vi "Reading HTML.vi"() -> ()   [LabVIEW 2024]
uses:
  <vilib>/httpClient/POSTBuffer.vi
  <vilib>/httpClient/LabVIEWHTTPClient.lvlib
panel:
  out "headers 3":string
  out "body 3":string
  out "headers 2":string
  out "body 2":string
  in  "Pulse number 2":string="5"
  out "body":string="{\"message\":\"success\"}"
  out "headers":string="HTTP/1.1 200 OK\r\nTransfer-Encoding: chunked\r\n\r\n"
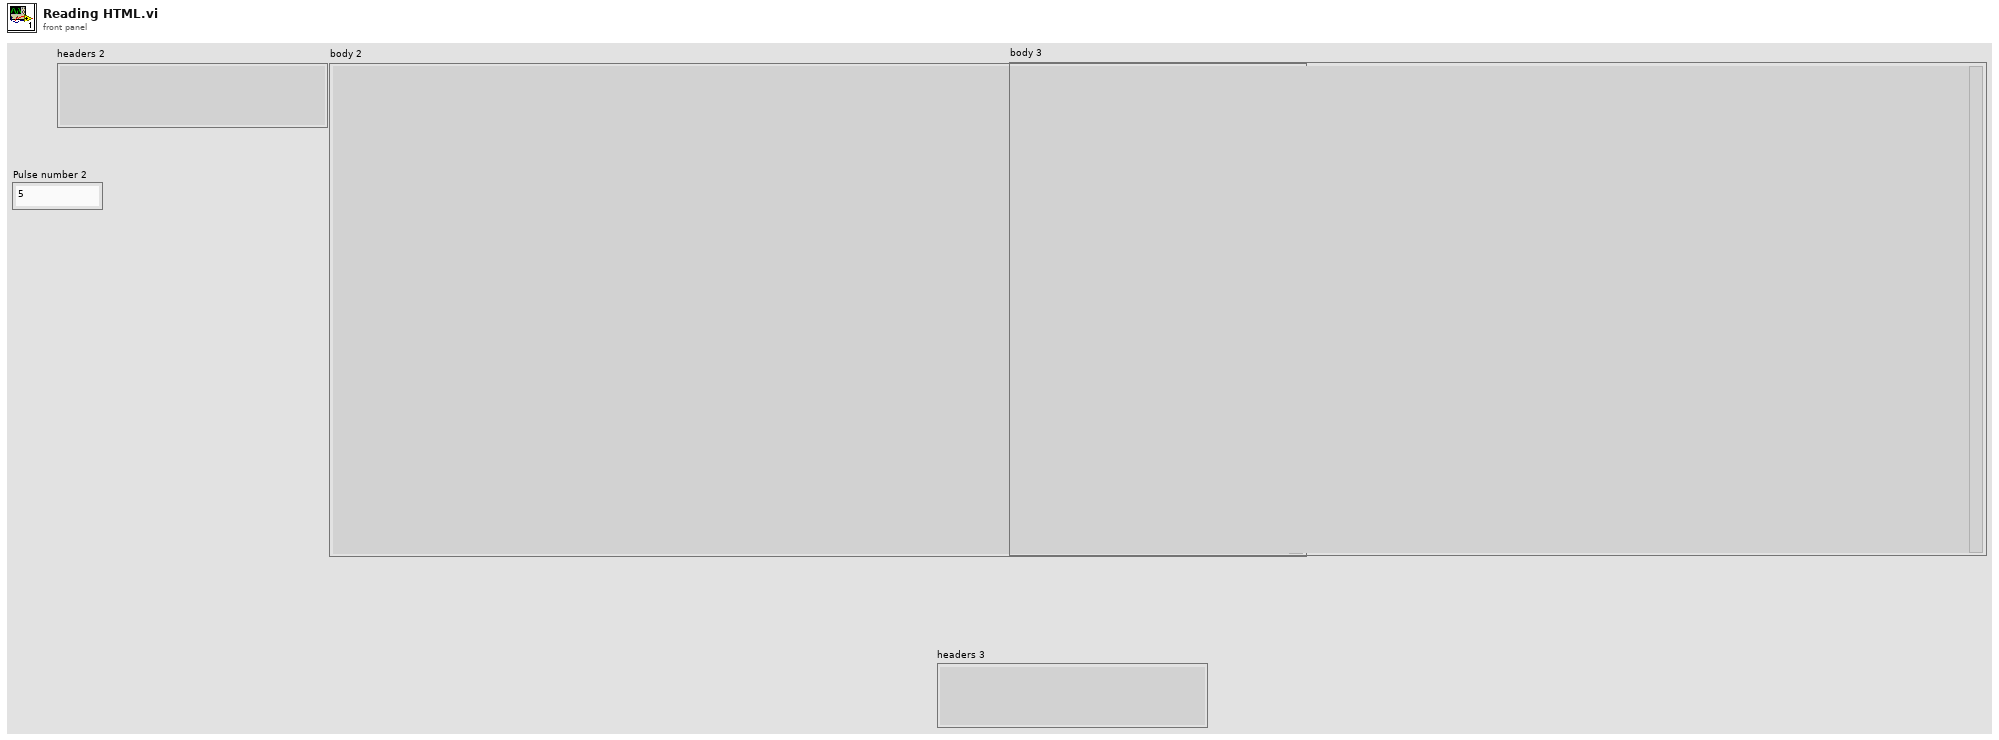
[diagram p1: front panel]
types:
  T1 = typedef "LabVIEWHTTPClient.lvlib/ClientHandle.ctl" = refnum<k1>
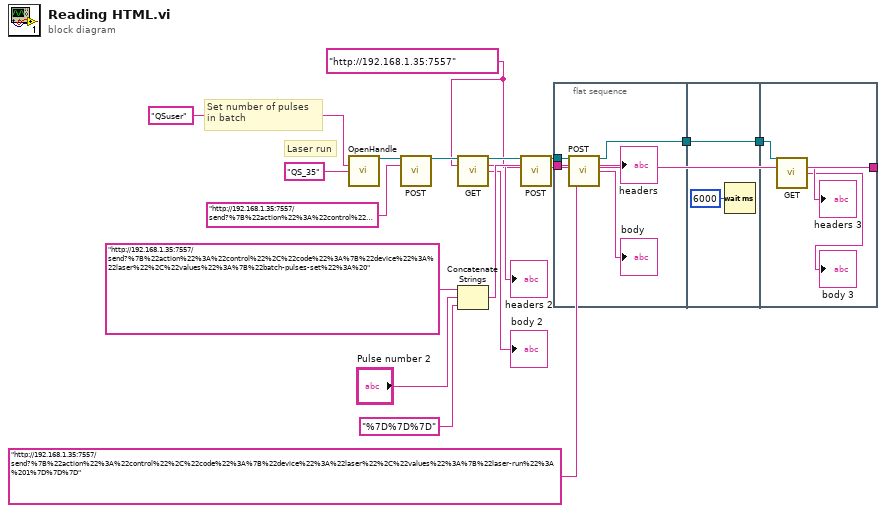
[diagram p0: block diagram]
diagram:
  w1 = "http://192.168.1.35:7557" ("url")
  # "Set number of pulses \nin batch"
  # "Laser run"
  n1 = call <vilib>:"OpenHandle.vi"("username"="QSuser", "password"="QS_35") -> ("client handle out"=w15:T1)  [unwired: 12 in, 1 out]
  n2 = call-poly <vilib>:"POST.vi"("client handle"=w15, "url"="http://192.168.1.35:7557/send?%7B%22action%22%3A%22control%22%2C%22code%22%3A%7B%22device%22%3A%22laser%22%2C%22values%22%3A%7B%22batch-mode%22%3A %201%7D%7D%7D") -> ("client handle out"=w5:T1)  [unwired: 10 in, 3 out]
  n3 = call <vilib>:"GET.vi"("client handle"=w5, "url"=w1) -> ("client handle out"=w4:T1, "headers"=→"headers 2":string, "body"=→"body 2":string)  [unwired: 10 in, 1 out]
  n4 = Concatenate Strings("http://192.168.1.35:7557/send?%7B%22action%22%3A%22control%22%2C%22code%22%3A%7B%22device%22%3A%22laser%22%2C%22values%22%3A%7B%22batch-pulses-set%22%3A%20" ("string"), "Pulse number 2", "%7D%7D%7D" ("string")) -> (w8:string)
  n5 = call-poly <vilib>:"POST.vi"("client handle"=w4, "url"=w8) -> ("client handle out"=w13:T1)  [unwired: 10 in, 3 out]
  n6 = flat-sequence {
    tunnel: w13 -> [w22]
    tunnel: "http://192.168.1.35:7557/send?%7B%22action%22%3A%22control%22%2C%22code%22%3A%7B%22device%22%3A%22laser%22%2C%22values%22%3A%7B%22laser-run%22%3A%201%7D%7D%7D" ("url") -> [w21]
    tunnel: [w18] -> w2
    tunnel: [w23] -> w3
    tunnel: w2 -> [w23]
    tunnel: w3 -> [w28]
    tunnel: w1 -> [w25]
    frame #0 {
      n7 = call-poly <vilib>:"POST.vi"("client handle"=w22, "url"=w21) -> ("client handle out"=w18:T1, "headers"=→"headers":string, "body"=→"body":string)  [unwired: 10 in, 1 out]
    }
    frame #1 {
      n8 = Wait (ms)(milliseconds to wait=u32 6000) -> ()  [unwired: 1 out]
    }
    frame #2 {
      n9 = call <vilib>:"GET.vi"("client handle"=w28, "url"=w25) -> ("headers"=→"headers 3":string, "body"=→"body 3":string)  [unwired: 10 in, 2 out]
    }
  }
